vi "DownKeyEvent.vi"() -> ()   [LabVIEW 2016]
panel:
  in  "Cluster":cluster{"Array":dbl[], "Array 2":dbl[]} {"Array 2" format="%#_6p"; "Array" format="%#_6p"}
  in  "Stop":bool
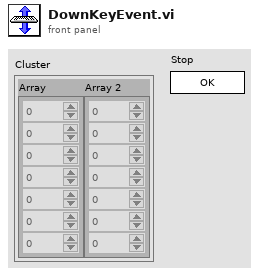
[diagram p1: front panel]
types:
  T1 = typedef "eventvkey.ctl" = enum16{"ASCII", "Enter", "Return", "Shift", "Ctrl", "Alt", "Cmd", "Opt", "Caps", "NumLock", "Clear", "Break", "Up", "Down", "Left", "Right", "Insert", "Delete", "Home", "End", "PageUp", "PageDown", "Escape", "Help", "Pause", "ScrollLock", "F1", "F2", "F3", "F4", "F5", "F6", "F7", "F8", "F9", "F10", "F11", "F12", "F13", "F14", "F15", "F16", "F17", "F18", "F19", "F20", "F21", "F22", "F23", "F24", "Play", "VolumeUp", "VolumeDown", "Mute", "Two Byte Char"}
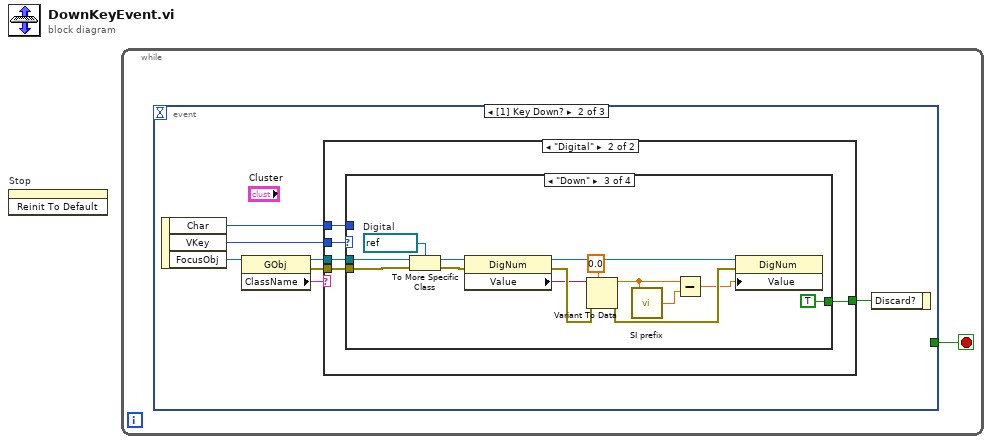
[diagram p0: block diagram]
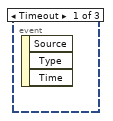
[diagram p2: hidden frame]
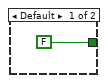
[diagram p3: hidden frame]
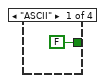
[diagram p4: hidden frame]
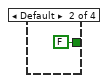
[diagram p5: hidden frame]
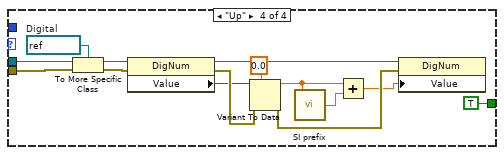
[diagram p6: hidden frame]
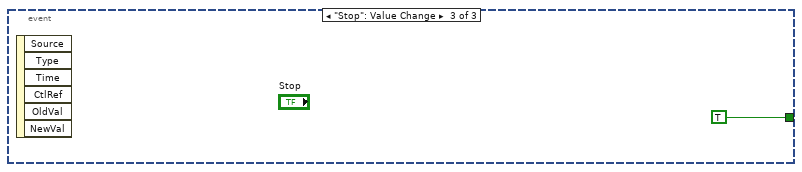
[diagram p7: hidden frame]
diagram:
  n1 = invoke on="Stop" class="Bool" method="Reinit To Default"() -> ()  [unwired: 3 in, 3 out]
  n2 = while {
    stop <- w1 stop-if-true
    n3 = event shown="[1] Key Down?" {
      selector: _ -> [_ _ _]
      dyn-events: _ -> [_ _ _]
      timeout: _ -> [_ _ _]
      tunnel: [_ _ TRUE] -> w1
      event Timeout {
        n4 = event-data() -> ()  [unwired: 1 in, 3 out]
      }
      event Key Down? {
        n5 = event-data() -> ("Char"=w2:i16, "VKey"=w6:T1, "FocusObj"=w8:refnum<vi>)  [unwired: 1 in]
        n6 = property class="GObj"(reference=w8) -> (reference out=w7:refnum<vi>, error out=w3:errorcluster, "ClassName"=w5:string)  [unwired: 1 in]
        n7 = case shown="\"Digital\"" w5 {
          tunnel: w7 -> [_ w14]
          tunnel: w6 -> [_ w13]
          tunnel: [FALSE ("x = y?") w10] -> w4
          tunnel: w3 -> [_ w12]
          tunnel: w2 -> [_ w11]
          frame Default {
          }
          frame "Digital" {
            n8 = case shown="\"Down\"" w13 {
              tunnel: w14 -> [_ _ w22 w35]
              tunnel: w12 -> [_ _ w21 w34]
              tunnel: w11 -> [_ _ _ _]
              tunnel: [FALSE ("x = y?") FALSE ("x = y?") TRUE ("x = y?") TRUE ("x = y?")] -> w10
              frame "ASCII" {
              }
              frame Default {
              }
              frame "Down" {
                w23 = refnum<vi> refnum  # Digital
                n9 = To More Specific Class(target class=w23, reference=w22, error in=w21) -> (specific class reference=w17:refnum<vi>, error out=w28:errorcluster)
                n10 = property class="DigNum"(reference=w17, error in=w28) -> (reference out=w27:refnum<vi>, error out=w29:errorcluster, "Value"=w25:variant)
                n11 = Variant To Data(error in=w29, type=0.0, Variant=w25) -> (data=w19:dbl, error out=w30:errorcluster)
                n12 = call "SI prefix.vi"("Numeric"=w19) -> ("Answer"=w18:dbl)
                n13 = Subtract(x=w19, y=w18) -> (x-y=w26:dbl)
                n14 = property class="DigNum"(reference=w27, error in=w30, "Value"=w26) -> ()  [unwired: 2 out]
              }
              frame "Up" {
                w37 = refnum<vi> refnum  # Digital
                n15 = To More Specific Class(target class=w37, reference=w35, error in=w34) -> (specific class reference=w36:refnum<vi>, error out=w42:errorcluster)
                n16 = property class="DigNum"(reference=w36, error in=w42) -> (reference out=w41:refnum<vi>, error out=w43:errorcluster, "Value"=w39:variant)
                n17 = Variant To Data(error in=w43, type=0.0, Variant=w39) -> (data=w32:dbl, error out=w44:errorcluster)
                n18 = call "SI prefix.vi"("Numeric"=w32) -> ("Answer"=w31:dbl)
                n19 = Add(x=w32, y=w31) -> (x+y=w40:dbl)
                n20 = property class="DigNum"(reference=w41, error in=w44, "Value"=w40) -> ()  [unwired: 2 out]
              }
            }
          }
        }
        n21 = event-data("Discard?"=w4) -> ()  [unwired: 1 in, 1 out]
      }
      event "Stop": Value Change {
        n22 = event-data() -> ()  [unwired: 1 in, 6 out]
      }
    }
  }
